vi "Vision_fullscreenwin_test.vi"(11 "Refnum in":T1="cam1") -> (0 "error out":errorcluster, 1 "Image (duplicate)":T3, 3 "Refnum out":T1, 4 "Center Point":T2)   [LabVIEW 2017]
doc: "This VI configures a USB camera for frame grabbing, and sets up the first image with the Traditional MeanShift tracking algorithm. Select the center point of the image, and place a rectangle around the region of interest to set up tracking."
uses:
  <vilib>/userdefined/High Color/IMAQdx.ctl
  <vilib>/vision/Image Controls.llb/IMAQ Image.ctl
  <vilib>/vision/driver/NI_Vision_Acquisition_Software.lvlib
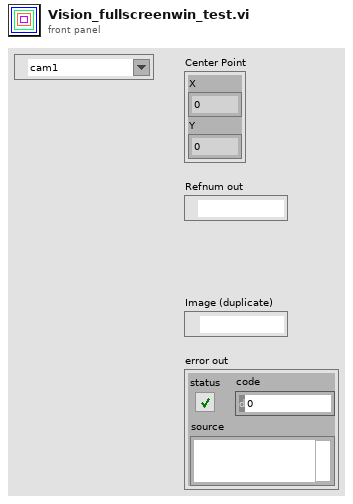
[diagram p1: front panel]
types:
  T1 = typedef "IMAQdx.ctl" = refnum<k21>
  T2 = typedef "IMAQ Point" = cluster{"X":sgl, "Y":sgl}
  T3 = typedef "IMAQ Image.ctl" = refnum<image>
  T4 = typedef "Image Type" = u32
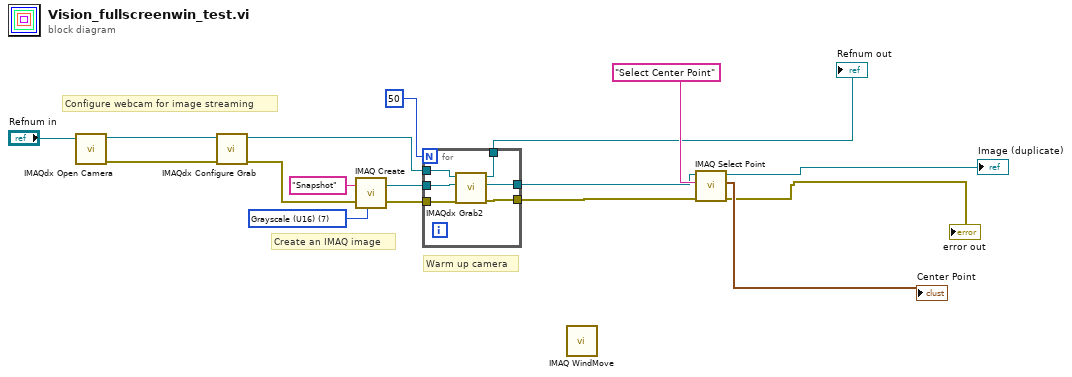
[diagram p0: block diagram]
diagram:
  w5 = T4 7 items=["Grayscale (U8)", "Grayscale (I16)", "Grayscale (SGL)", "Complex (CSG)", "RGB (U32)", "HSL (U32)", "RGB (U64)", "Grayscale (U16)"] ("Image Type")
  # "Warm up camera"
  # "Create an IMAQ image"
  # "Configure webcam for image streaming"
  n1 = call <vilib>:"IMAQdx Open Camera.vi"("Session In"="Refnum in") -> ("error out"=w7:errorcluster, "Session Out"=w6:T1)  [unwired: 9 in]
  n2 = call <vilib>:"IMAQdx Configure Grab.vi"("error in"=w7, "Session In"=w6) -> ("error out"=w8:errorcluster, "Session Out"=w10:T1)  [unwired: 8 in]
  n3 = call "IMAQ Create"("Image Name"="Snapshot", "Image Type"=w5, "error in (no error)"=w8) -> ("New Image"=w11:T3, "error out"=w12:errorcluster)  [unwired: 2 in]
  n4 = for {
    N: 50 -> [_]
    tunnel: w10 -> [w23]
    tunnel: w11 -> [w22]
    tunnel: w12 -> [w21]
    tunnel: [w20] -> w3
    tunnel: [w19] -> w14
    tunnel: [w18] -> w13
    n5 = call <vilib>:"IMAQdx Grab2.vi"("error in"=w21, "Image In"=w22, "Session In"=w23) -> ("error out"=w20:errorcluster, "Image Out"=w19:T3, "Session Out"=w18:T1)  [unwired: 5 in, 1 out]
  }
  "Refnum out" <- w13
  n6 = call "IMAQ WindMove"() -> ()  [unwired: 5 in, 2 out]
  n7 = call "IMAQ Select Point"("error in (no error)"=w3, "Prompt"="Select Center Point", "Image In"=w14) -> ("error out"=→"error out":errorcluster, "Point"=→"Center Point":T2, "Image Out (duplicate)"=→"Image (duplicate)":T3)  [unwired: 5 in, 1 out]
